vi "Set Destination.vi"(1 "Initial Position":dbl[](array[numeric]), 2 "Scores with Matching":cluster{"Z":dbl[], "Score":sgl[]}) -> (0 "Configuration":T1 {"Manual Control"."Z step" scale=0.1..10.0; "Manual Control"."XY Step" scale=0.1..1000.0})   [LabVIEW 2014]
uses:
  XYZ Stage/XYZ Config.ctl
  XYZ Stage/XYZ Connection Settings.ctl
  XYZ Stage/XYZ Stage Control.ctl
  XYZ Stage/XYZ Coordinate Control.ctl
panel:
  # "LICENSED MATERIALS – PROPERTY OF IBM\nCopyright IBM Corp. 2016,\nALL RIGHTS RESERVED"
  # "XY"
  # "Z"
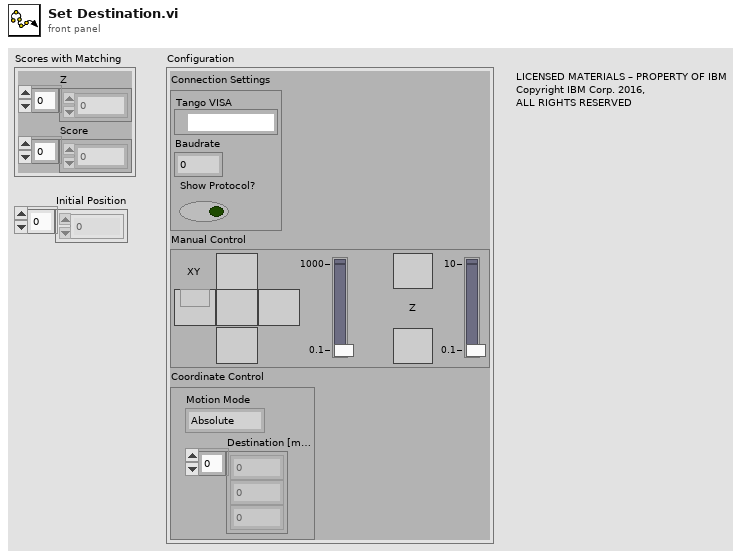
[diagram p1: front panel]
types:
  T1 = typedef "XYZ Config.ctl" = cluster{"Connection Settings":T2, "Manual Control":T3, "Coordinate Control":T4}
  T2 = typedef "XYZ Connection Settings.ctl" = cluster{"Tango VISA":refnum<visa-resource-name>, "Baudrate":i32, "Show Protocol?":bool}
  T3 = typedef "XYZ Stage Control.ctl" = cluster{"North":bool, "South":bool, "West":bool, "East":bool, "Up":bool, "Down":bool, "Stop":bool, "XY Step":dbl, "Z step":dbl}
  T4 = typedef "XYZ Coordinate Control.ctl" = cluster{"Motion Mode":enum16{"Absolute", "Relative"}, "Destination [mm]":dbl[]}
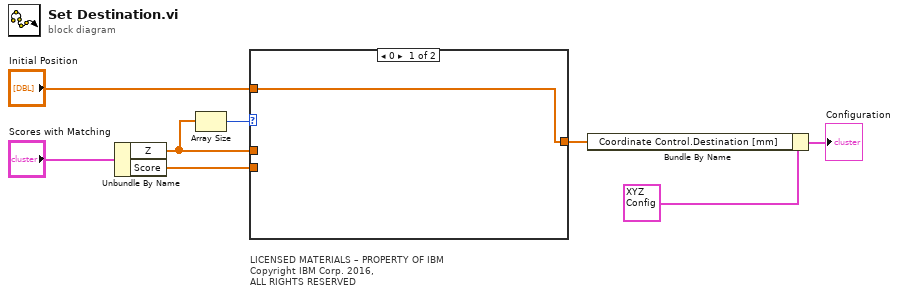
[diagram p0: block diagram]
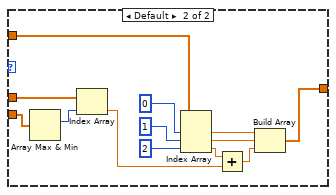
[diagram p2: hidden frame]
diagram:
  # "LICENSED MATERIALS – PROPERTY OF IBM\nCopyright IBM Corp. 2016,\nALL RIGHTS RESERVED"
  n1 = Unbundle By Name("Scores with Matching") -> ("Z"=w2:dbl[], "Score"=w4:sgl[])
  n2 = Array Size(array=w2) -> (size(s)=w1:i32)
  n3 = case shown="0" w1 {
    tunnel: [w9 w22] -> w6
    tunnel: "Initial Position" -> [w9 w21]
    tunnel: w4 -> [_ w15]
    tunnel: w2 -> [_ w14]
    frame 0 {
    }
    frame Default {
      n4 = Array Max & Min(array=w15) -> (max index (indices)=w16:i32)  [unwired: 3 out]
      n5 = Index Array(array=w14, index=w16) -> (element=w11:dbl)
      n6 = Index Array(array=w21, index #1=0 ("index"), index #2=1 ("index"), index #3=2 ("index")) -> (element #1=w19:dbl, element #2=w20:dbl, element #3=w12:dbl)
      n7 = Add(x=w12, y=w11) -> (x+y=w13:dbl)
      n8 = Build Array(w19, w20, w13) -> (w22:dbl[])
    }
  }
  n9 = Bundle By Name(cluster=T1 {"Connection Settings"={"Tango VISA"="", "Baudrate"=57600, "Show Protocol?"=FALSE}, "Manual Control"={"North"=FALSE, "South"=FALSE, "West"=FALSE, "East"=FALSE, "Up"=FALSE, "Down"=FALSE, "Stop"=FALSE, "XY Step"=0.0, "Z step"=0.0}, "Coordinate Control"={"Motion Mode"=enum."Absolute", "Destination [mm]"=[]}} ("Configuration"), "Coordinate Control.Destination [mm]"=w6) -> (→"Configuration":T1)
